vi "TOF ONS.vi"(9 "Delay (ms)":u32=500, 10 "Input":bool) -> (2 "Output":bool)   [LabVIEW 2013]
doc: "The TOF ONS, when given a True input, will immediately output True for one pulse, then revert back to False. When the input reverts back to False, the output will wait for the specified delay to elapse before resetting and allowing an input again."
panel:
  out "Last State":bool
  in  "Delay_TOF":T1={"Timer_States"=enum."Input_False_Timing", "Delay-Done_Time"=0}
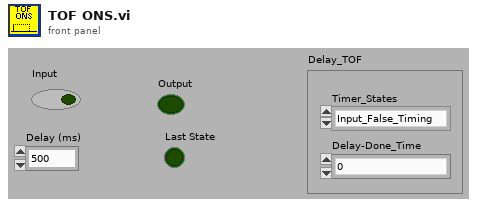
[diagram p1: front panel]
types:
  T1 = cluster{"Timer_States":enum16{"Input_True", "Input_False_Timing", "Input_False_Timing_Complete"}, "Delay-Done_Time":u32}
  T2 = enum16{"Input_True", "Input_False_Timing", "Input_False_Timing_Complete"}
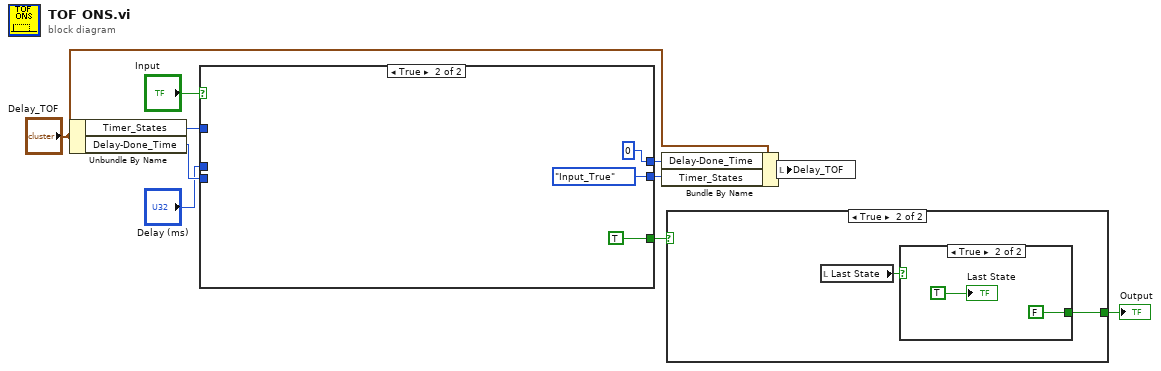
[diagram p0: block diagram]
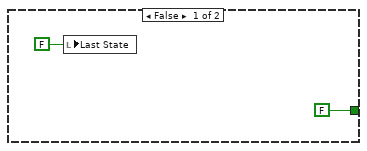
[diagram p2: hidden frame]
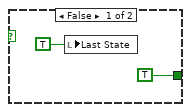
[diagram p3: hidden frame]
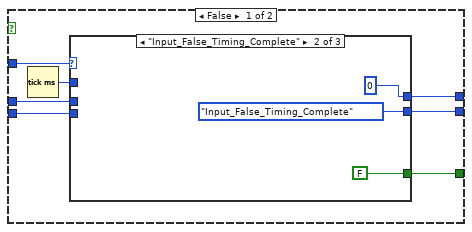
[diagram p4: hidden frame]
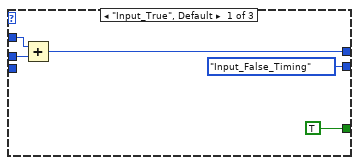
[diagram p5: hidden frame]
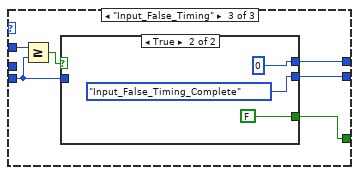
[diagram p6: hidden frame]
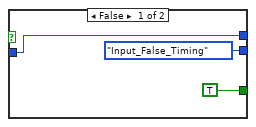
[diagram p7: hidden frame]
diagram:
  n1 = Unbundle By Name("Delay_TOF") -> ("Timer_States"=w6:T2, "Delay-Done_Time"=w9:u32)
  n2 = case shown="True" "Input" {
    tunnel: [w14 TRUE] -> w1
    tunnel: [w15 T2."Input_True" ("Timer_States")] -> w3
    tunnel: [w16 u32 0 ("Delay-Done_Time")] -> w4
    tunnel: w9 -> [w11 _]
    tunnel: w6 -> [w13 _]
    tunnel: "Delay (ms)" -> [w12 _]
    frame False {
      n3 = Tick Count (ms)() -> (millisecond timer value=w17:u32)
      n4 = case shown="\"Input_False_Timing_Complete\"" w13 {
        tunnel: w17 -> [w21 _ w31]
        tunnel: [w19 u32 0 ("Delay-Done_Time") w26] -> w16
        tunnel: [T2."Input_False_Timing" ("Timer_States") T2."Input_False_Timing_Complete" ("Timer_States") w29] -> w15
        tunnel: [TRUE FALSE w28] -> w14
        tunnel: w12 -> [w20 _ _]
        tunnel: w11 -> [_ _ w27]
        frame "Input_True", Default {
          n5 = Add(x=w21, y=w20) -> (x+y=w19:u32)
        }
        frame "Input_False_Timing_Complete" {
        }
        frame "Input_False_Timing" {
          n6 = Greater Or Equal?(x=w31, y=w27) -> (x >= y?=w30:bool)
          n7 = case shown="True" w30 {
            tunnel: [T2."Input_False_Timing" ("Timer_States") T2."Input_False_Timing_Complete" ("Timer_States")] -> w29
            tunnel: [TRUE FALSE] -> w28
            tunnel: w27 -> [w32 _]
            tunnel: [w32 u32 0 ("Delay-Done_Time")] -> w26
            frame False {
            }
            frame True {
            }
          }
        }
      }
    }
    frame True {
    }
  }
  n8 = Bundle By Name(cluster="Delay_TOF", "Delay-Done_Time"=w4, "Timer_States"=w3) -> (w8:T1)
  n9 = case shown="True" w1 {
    tunnel: [FALSE ("One-Shot Output") w44] -> w2
    frame False {
      n10 = local write "Last State"(FALSE ("Last State")) -> ()
    }
    frame True {
      n11 = local read "Last State"() -> (w43:bool)
      n12 = case shown="True" w43 {
        tunnel: [TRUE ("One-Shot Output") FALSE ("One-Shot Output")] -> w44
        frame False {
          n13 = local write "Last State"(TRUE ("Last State")) -> ()
        }
        frame True {
          "Last State" <- TRUE ("Last State")
        }
      }
    }
  }
  "Output" <- w2
  n14 = local write "Delay_TOF"(w8) -> ()
